vi "Escape String2.vi"(11 "input":string) -> (3 "output":string)   [LabVIEW 2017]
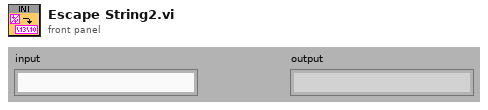
[diagram p1: front panel]
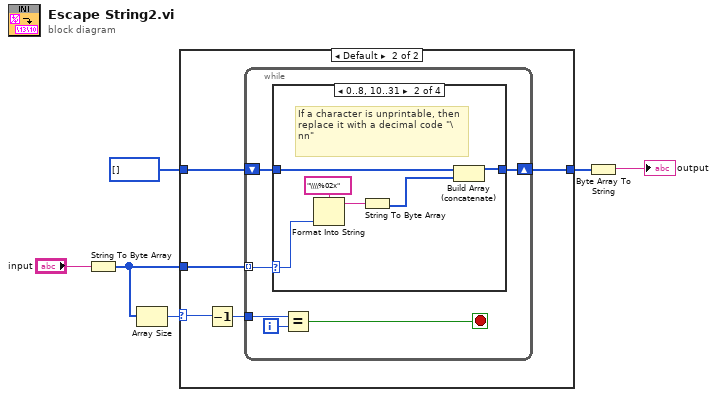
[diagram p0: block diagram]
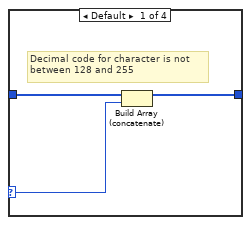
[diagram p3: hidden frame]
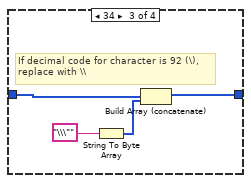
[diagram p4: hidden frame]
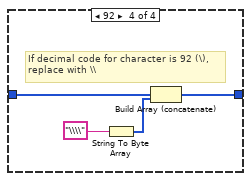
[diagram p5: hidden frame]
diagram:
  n1 = String To Byte Array(string="input") -> (unsigned byte array=w5:u8[])
  n2 = Array Size(array=w5) -> (size(s)=w3:i32)
  n3 = case shown="Default" w3 {
    selector: w3 -> [_ w8]
    tunnel: u8[] [] -> [_ w12]
    tunnel: w5 -> [w7 w11]
    tunnel: [w7 w9] -> w4
    frame 0 {
    }
    frame Default {
      n4 = Decrement(x=w8) -> (x-1=w10:i32)
      n5 = while {
        tunnel: w11 -> [w15] mode=indexing
        shift-right: [w17] -> w9
        shift-left: w12 -> [w18]
        tunnel: w10 -> [w14]
        i -> [w16]
        stop <- w13 stop-if-true
        n6 = case shown="0..8, 10..31" w15 {
          selector: w15 -> [w19 w22 _ _]
          tunnel: w18 -> [w21 w27 w29 w34]
          tunnel: [w20 w26 w28 w33] -> w17
          frame Default {
            # "Decimal code for character is not \nbetween 128 and 255"
            n7 = Build Array (concatenate)(w21, w19) -> (w20:u8[])
          }
          frame 0..8, 10..31 {
            # "If a character is unprintable, then  replace it with a decimal code \"\\nn\""
            n8 = Format Into String(format string="\\\\%02x" ("Format String"), w22) -> (resulting string=w24:string)  [unwired: 2 in, 1 out]
            n9 = String To Byte Array(string=w24) -> (unsigned byte array=w23:u8[])
            n10 = Build Array (concatenate)(w27, w23) -> (w26:u8[])
          }
          frame 34 {
            # "If decimal code for character is 92 (\\),\nreplace with \\\\"
            n11 = String To Byte Array(string="\\\"" ("Format String")) -> (unsigned byte array=w30:u8[])
            n12 = Build Array (concatenate)(w29, w30) -> (w28:u8[])
          }
          frame 92 {
            # "If decimal code for character is 92 (\\),\nreplace with \\\\"
            n13 = String To Byte Array(string="\\\\" ("Format String")) -> (unsigned byte array=w32:u8[])
            n14 = Build Array (concatenate)(w34, w32) -> (w33:u8[])
          }
        }
        n15 = Equal?(x=w14, y=w16) -> (x = y?=w13:bool)
      }
    }
  }
  n16 = Byte Array To String(unsigned byte array=w4) -> (string=→"output":string)
